vi "TAT_Start.vi"(8 "error In":errorcluster) -> ()   [LabVIEW 2017]
uses:
  <vilib>/addons/database/Connection.llb/Conn ObjectReference.ctl
  Controls/Ass. Loop Control.ctl
  <vilib>/addons/database/Connection.llb/DB Tools Open Connec (Path).vi
  <vilib>/addons/database/NI_Database_API.lvlib
panel:
  out "CYCLE COUNT STATION 2":string caption="CYCLE COUNT"
  out "RESULT STATION 2":bool caption="RESULT"
  out "BARCODE STATION 2":string caption="BARCODE"
  out "CYCLE STATUS STATION 2":string caption="CYCLE STATUS"
  out "PLC":bool
  in  "Stop":bool
  out "error out":errorcluster
  out "CYCLE COUNT STATION 1":string caption="CYCLE COUNT"
  out "BARCODE STATION 1":string caption="BARCODE"
  out "RESULT STATION 1":bool caption="RESULT"
  out "VARIENT":string
  out "USER":string
  in  "ASS-Alarms":bool
  in  "T-Alarms":bool
  out "CYCLE STATUS STATION 1":string caption="CYCLE STATUS"
  out "DATE/TIME":string
  # "RBC ORVM- TRACEABILITY, SCANNING & BARCODE PRINTING"
  # "STATION 1"
  # "STATION 2"
  # "Nm"
  # "REMAINING SQL CODE TO WRITE"
  # "KAPSE SONS ROBOTICS\n& AUTOMATION"
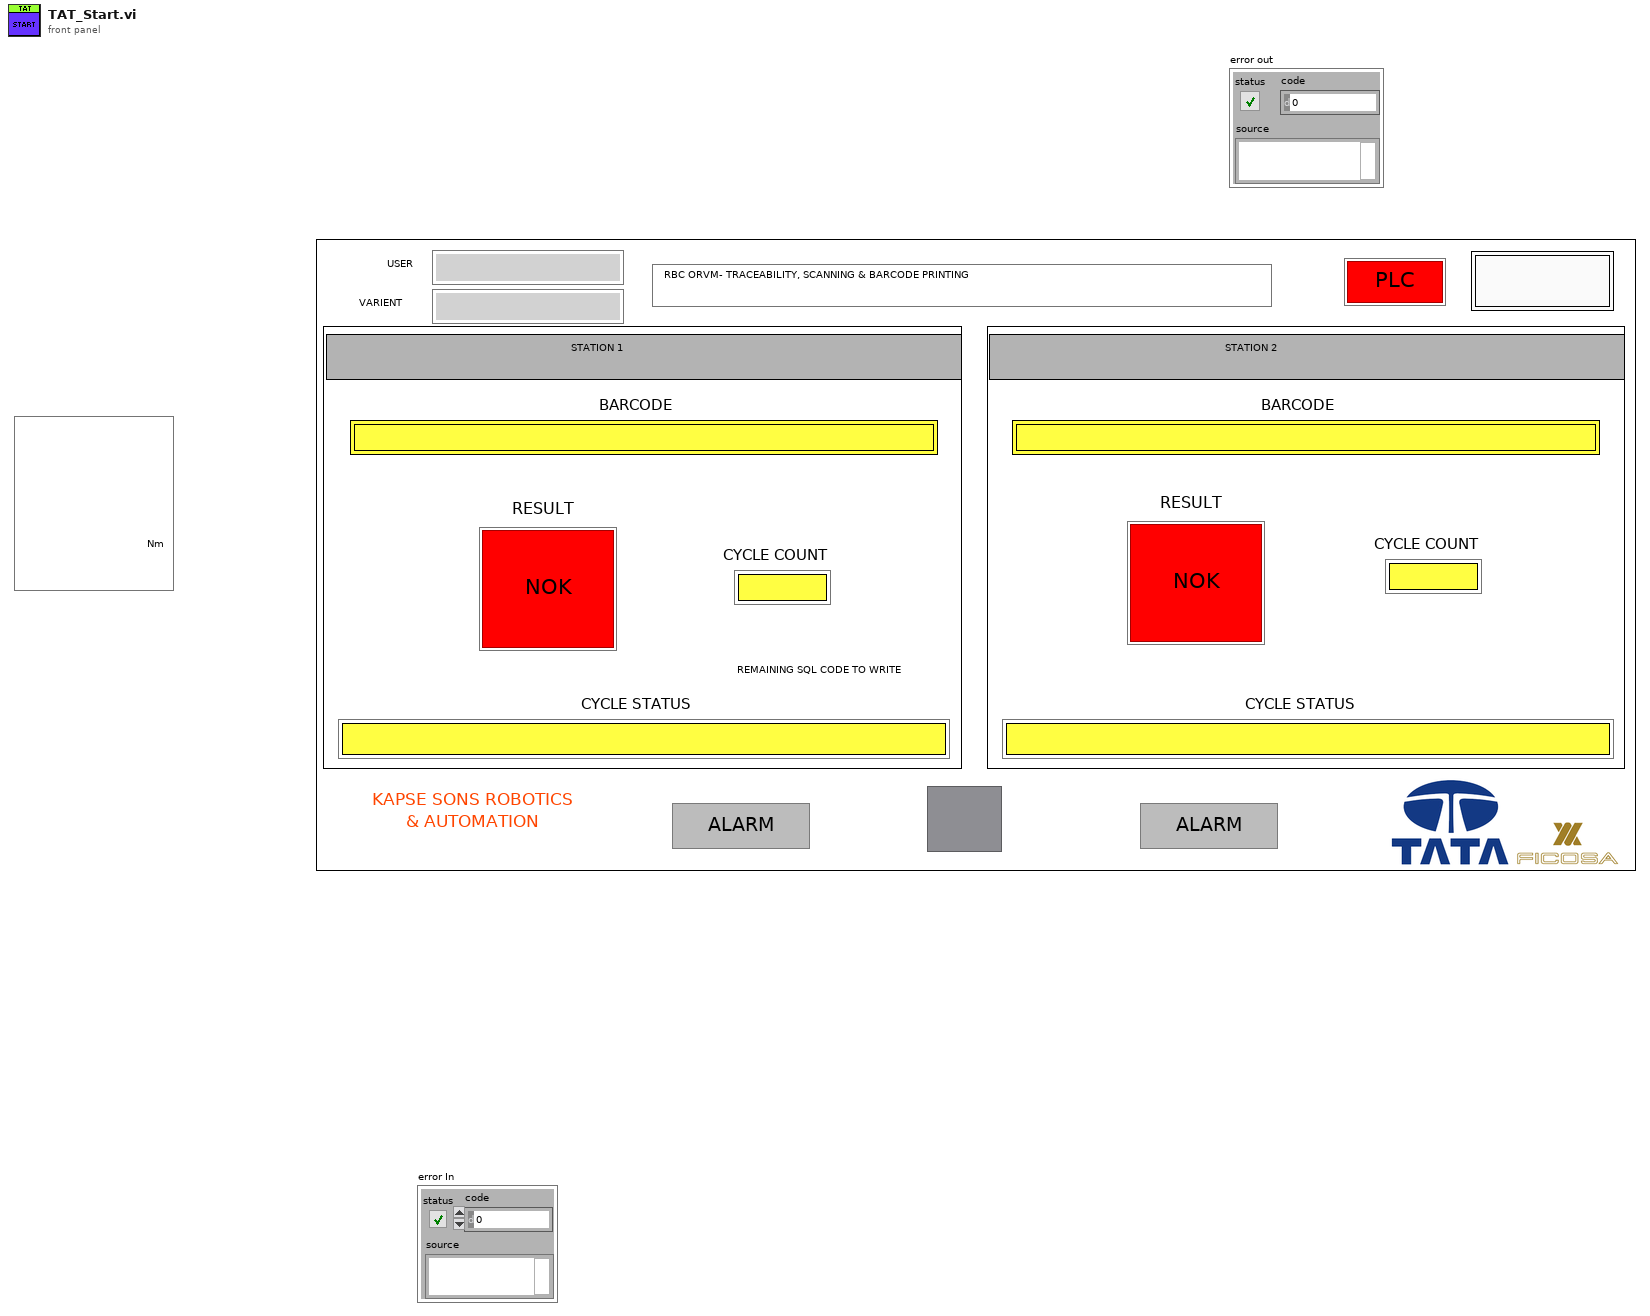
[diagram p1: front panel]
types:
  T1 = typedef "Ass. Loop Control.ctl" = enum16{"Cluster_update", "Waiting_for_scan", "barcode scan", "Int", "SaveReport ", "Barcode Print", "Start Cycle", "Wait", "Cycle End", "Stop"}
  T2 = typedef "NI_Database_API.lvlib/Conn ObjectReference.ctl" = refnum<k1>
  T3 = cluster{"Varient number":i32, "Varient name":string, "connection ID":refnum<k5>, "connection reference":T2, "Varient_Counter":u16}
  T4 = cluster{"Varient number":u16, "Varient name":string, "Barcode prefix":string, "connection ID":refnum<k5>, "connection reference":T2, "Batch_Size":u16}
  T5 = cluster{"seconds since 1Jan1904":timestamp, "Varient name":string, "BARCODE STATION 1":string, "table":string, "table":string}
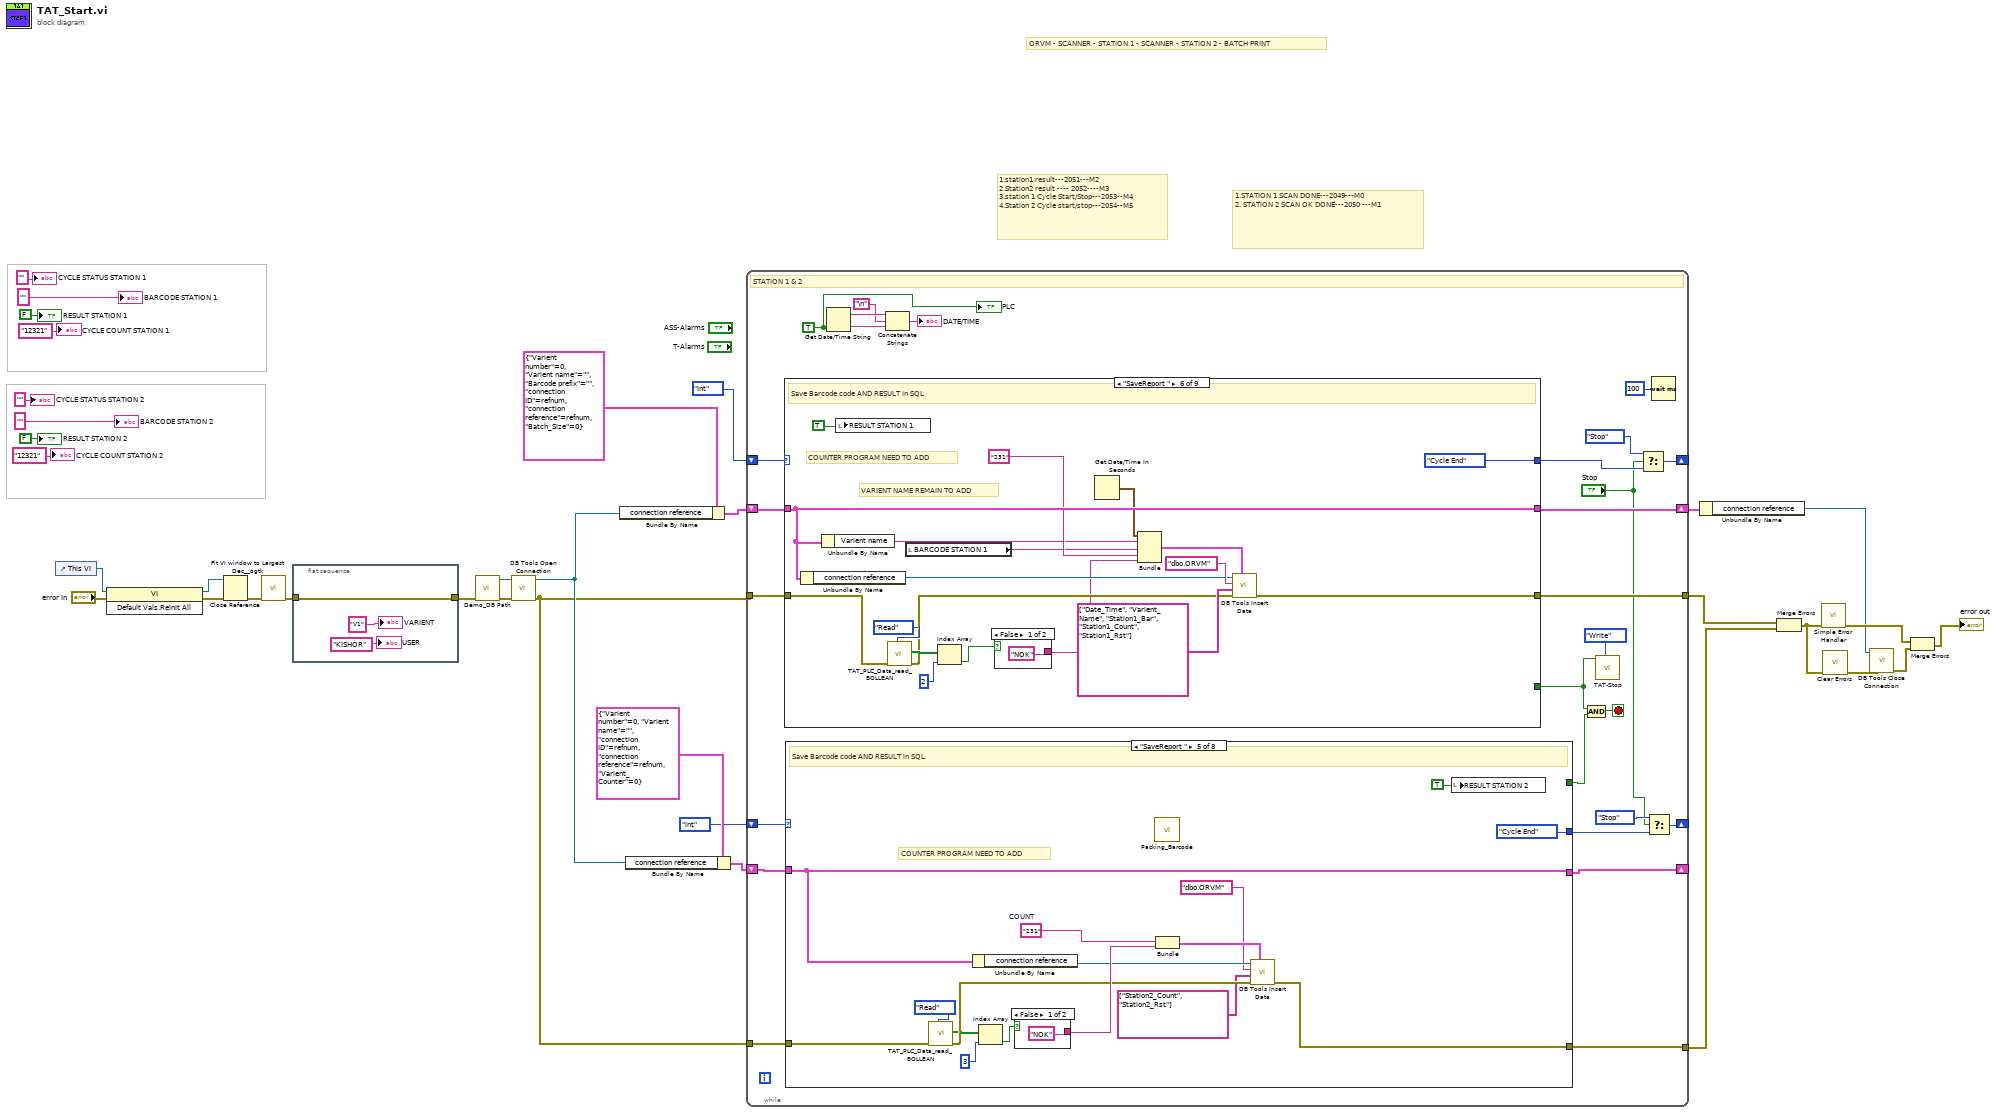
[diagram p0: block diagram]
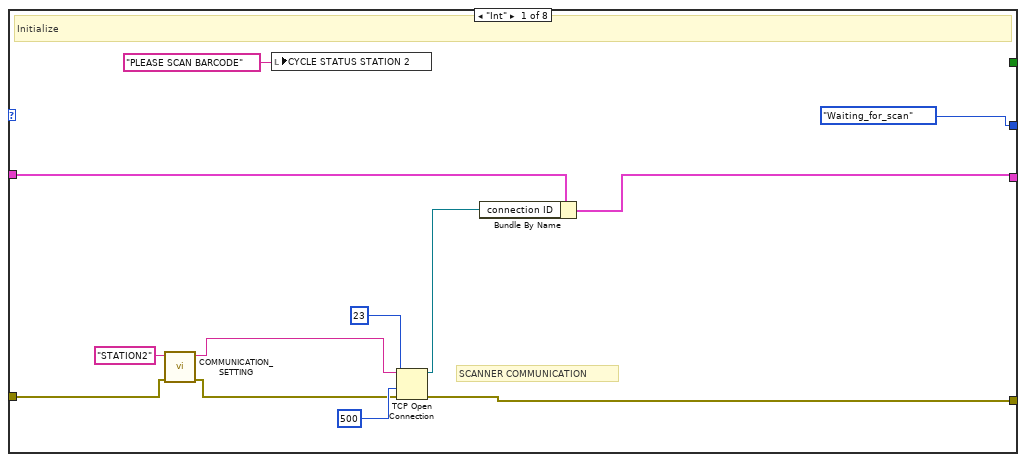
[diagram p2: hidden frame]
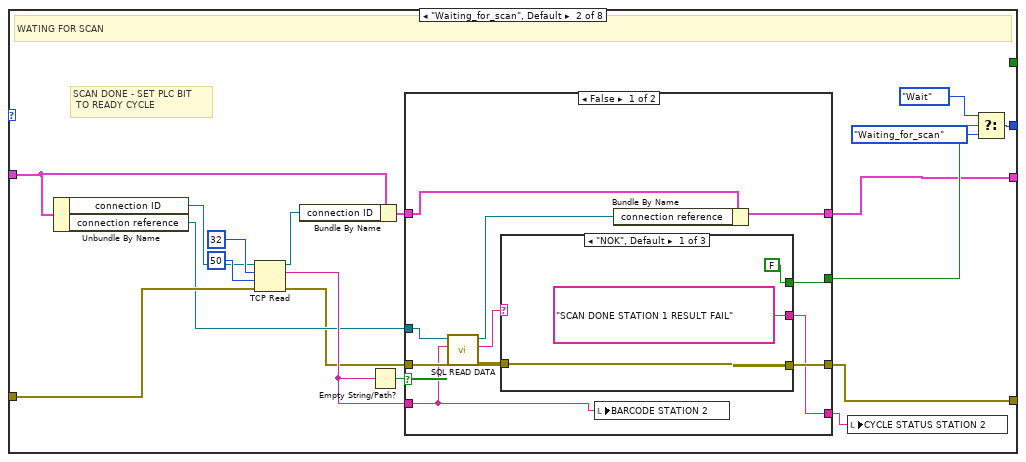
[diagram p3: hidden frame]
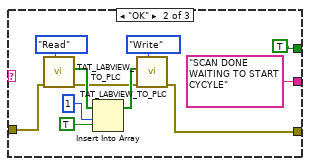
[diagram p4: hidden frame]
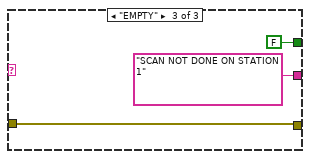
[diagram p5: hidden frame]
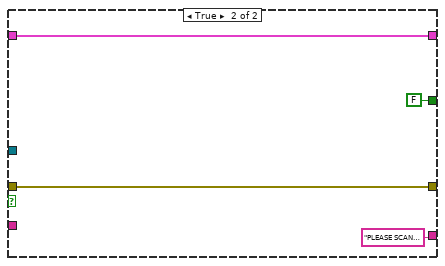
[diagram p6: hidden frame]
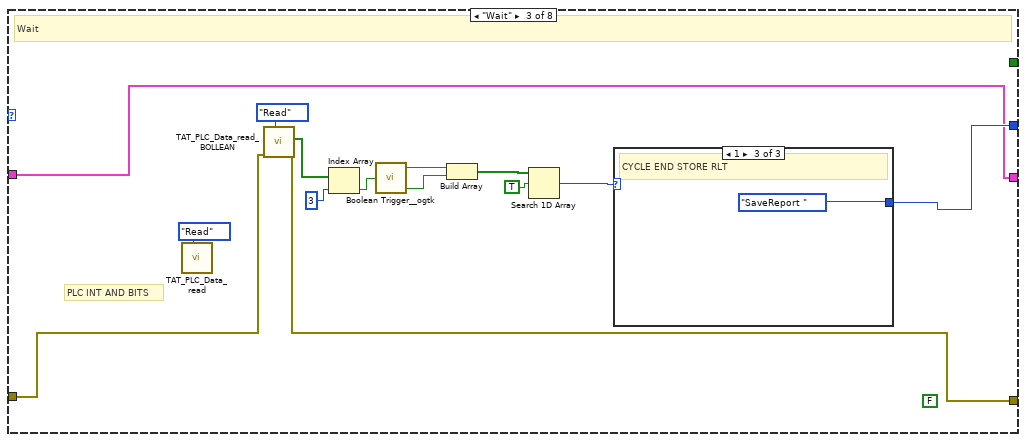
[diagram p7: hidden frame]
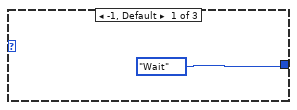
[diagram p8: hidden frame]
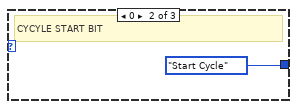
[diagram p9: hidden frame]
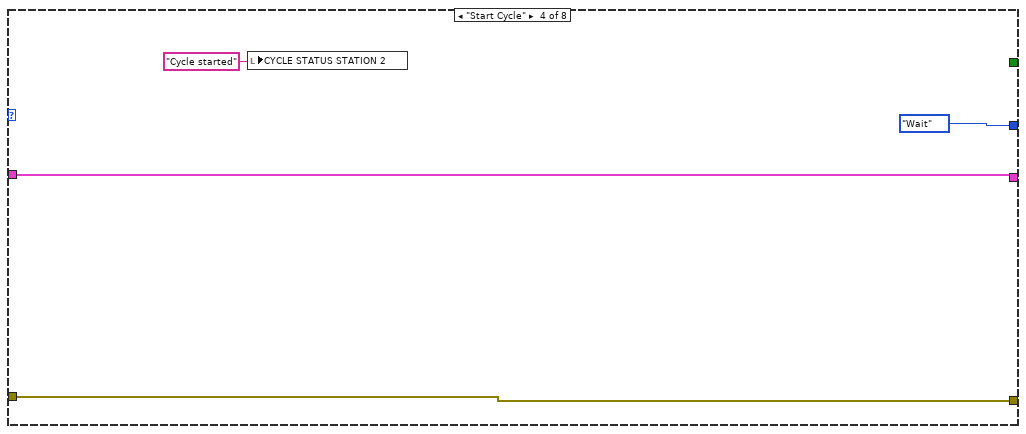
[diagram p10: hidden frame]
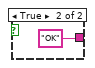
[diagram p11: hidden frame]
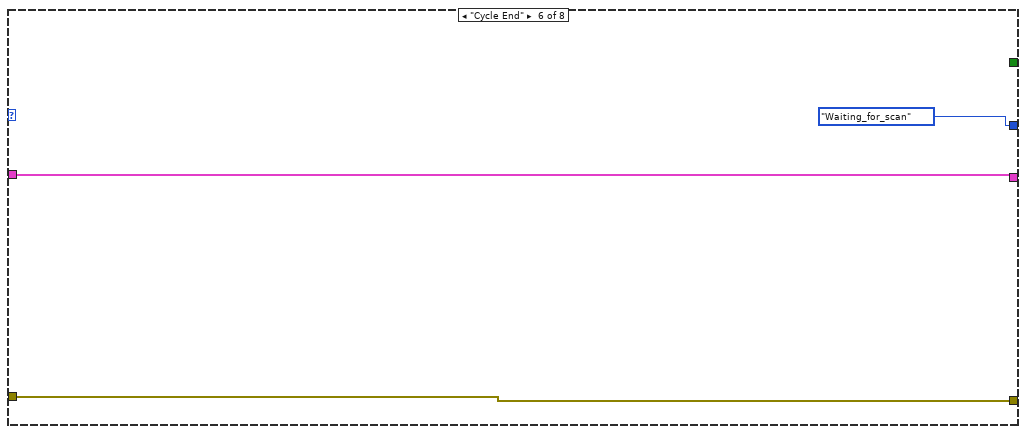
[diagram p12: hidden frame]
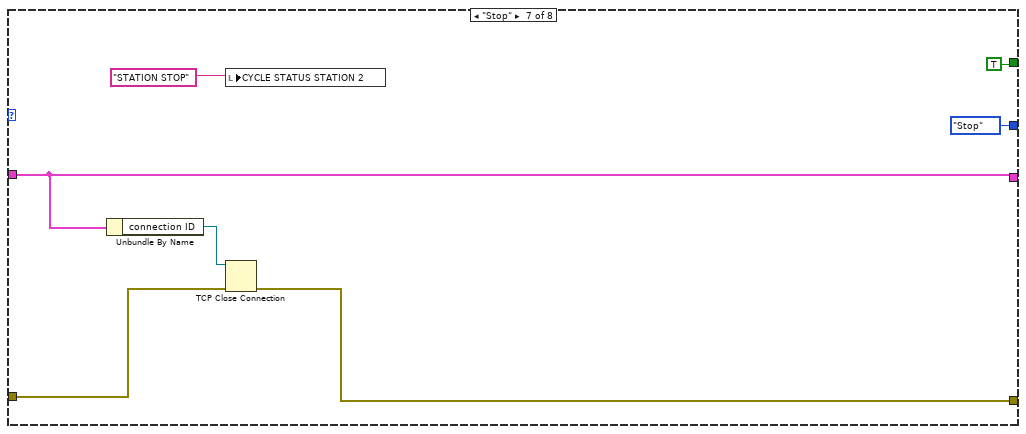
[diagram p13: hidden frame]
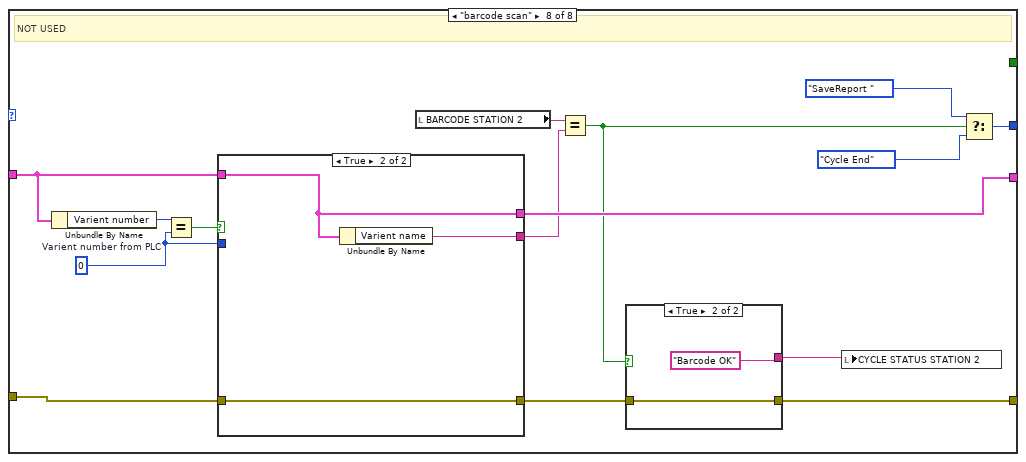
[diagram p14: hidden frame]
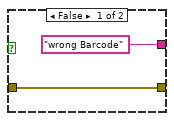
[diagram p15: hidden frame]
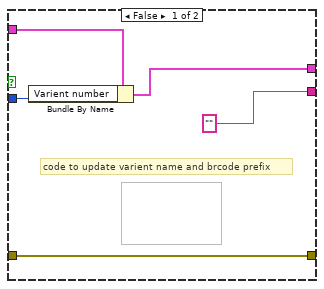
[diagram p16: hidden frame]
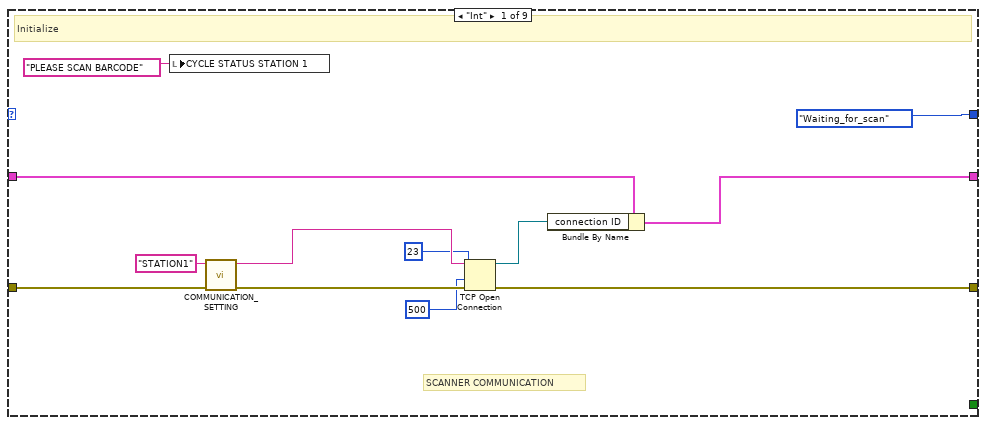
[diagram p17: hidden frame]
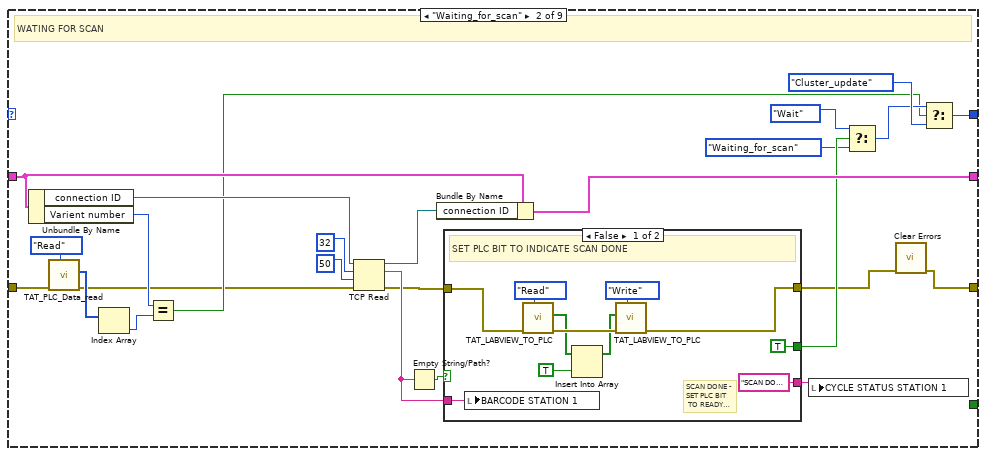
[diagram p18: hidden frame]
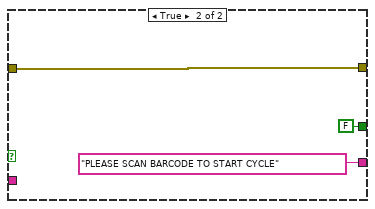
[diagram p19: hidden frame]
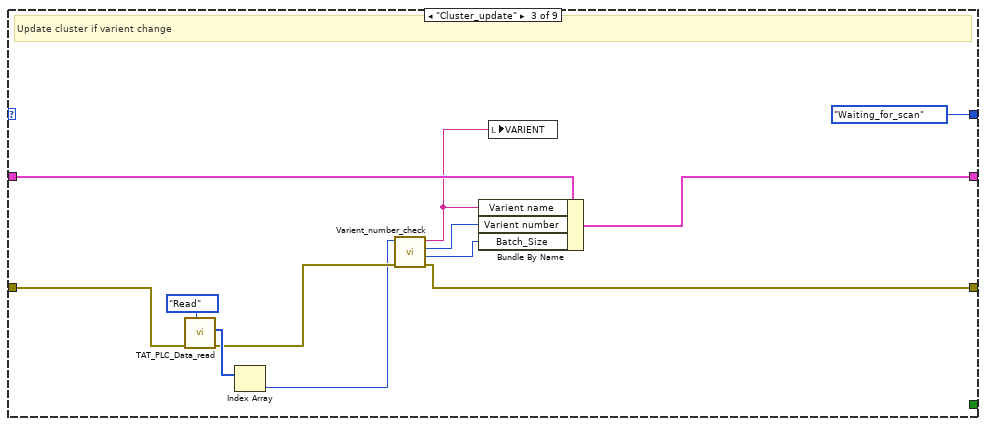
[diagram p20: hidden frame]
diagram:
  # "1.STATION 1 SCAN DONE---2049---M0\n2. STATION 2 SCAN OK DONE---2050 ---M1"
  # "1.station1 result---2051---M2\n2.Station2 result ---- 2052----M3\n3.station 1 Cycle Start/Stop---2053--M4\n4.Station 2 Cycle start/stop---2054--M5"
  # "ORVM - SCANNER - STATION 1 - SCANNER - STATION 2 - BATCH PRINT"
  n1 = control-ref of="This VI"() -> (w34:refnum<vi>)
  n2 = invoke class="VI" method="Default Vals.Reinit All"(reference=w34, error in="error In") -> (reference out=w31:refnum<vi>, error out=w32:errorcluster)  [unwired: 1 in, 1 out]
  n3 = Close Reference(reference=w31, error in (no error)=w32) -> (error out=w30:errorcluster)
  n4 = call <userlib>:"Fit VI window to Largest Dec__ogtk.vi"("error in (no error)"=w30) -> ("error out"=w29:errorcluster)  [unwired: 5 in, 1 out]
  n5 = flat-sequence {
    tunnel: [w37] -> w12
    tunnel: w29 -> [w37]
    frame #0 {
      "USER" <- "KISHOR"
      "VARIENT" <- "V1"
    }
  }
  n6 = call "Demo_DB Path.vi"("error in"=w12) -> ("error out"=w10:errorcluster, "DB Path"=w11:path)  [unwired: 9 in]
  n7 = call-poly <vilib>:"DB Tools Open Connection.vi"("error in (no error)"=w10, "connection information"=w11) -> ("error out"=w1:errorcluster, "connection reference"=w9:T2)  [unwired: 6 in]
  n8 = Bundle By Name(cluster=T4 {"Varient number"=0, "Varient name"="", "Barcode prefix"="", "connection ID"=refnum, "connection reference"=refnum, "Batch_Size"=0}, "connection reference"=w9) -> (w22:T4)
  n9 = Bundle By Name(cluster=T3 {"Varient number"=0, "Varient name"="", "connection ID"=refnum, "connection reference"=refnum, "Varient_Counter"=0}, "connection reference"=w9) -> (w20:T3)
  n10 = while {
    tunnel: w1 -> [w59]
    shift-right: [w58] -> _
    shift-left: Ass._Loop_Control."Int" ("Enum") -> [w64]
    shift-right: [w62] -> w3
    shift-left: w22 -> [w61]
    tunnel: [w60] -> w24
    tunnel: w1 -> [w50]
    tunnel: [w49] -> w13
    shift-right: [w46] -> _
    shift-left: w20 -> [w48]
    shift-right: [w43] -> _
    shift-left: Ass._Loop_Control."Int" ("Enum") -> [w47]
    stop <- w41 stop-if-true
    w51 = TRUE ("want seconds? (F)")
    # "STATION 1 & 2"
    n11 = case shown="\"SaveReport \"" w64 {
      tunnel: [Ass._Loop_Control."Waiting_for_scan" ("Enum") w218 Ass._Loop_Control."Waiting_for_scan" ("Enum") w273 Ass._Loop_Control."Wait" ("Enum") Ass._Loop_Control."Cycle End" ("Enum") Ass._Loop_Control."Waiting_for_scan" ("Enum") Ass._Loop_Control."Stop" ("Enum") w323] -> w57
      tunnel: [w206 w232 w257 w275 w287 w304 w311 w314 w329] -> w62
      tunnel: w61 -> [w207 w233 w258 w275 w287 w304 w311 w314 w330]
      tunnel: [_ _ _ FALSE _ _ _ TRUE _] -> w38
      tunnel: [w203 w226 w264 w267 w284 w299 w310 w315 w321] -> w60
      tunnel: w59 -> [w204 w223 w261 w268 w284 w288 w310 w316 w332]
      frame "Int" {
        # "SCANNER COMMUNICATION"
        # "Initialize"
        n12 = local write "CYCLE STATUS STATION 1"("PLEASE SCAN BARCODE" ("Cycle Status")) -> ()
        n13 = call "COMMUNICATION_SETTING.vi"("error in"=w204, "STATION"="STATION1") -> ("error out"=w212:errorcluster, "COM"=w210:string)  [unwired: 8 in]
        n14 = TCP Open Connection(address=w210, remote port or service name=u16 23, timeout ms (60000)=500, error in (no error)=w212) -> (connection ID=w205:refnum<k5>, error out=w203:errorcluster)  [unwired: 1 in]
        n15 = Bundle By Name(cluster=w207, "connection ID"=w205) -> (w206:T4)
      }
      frame "Waiting_for_scan" {
        # "WATING FOR SCAN"
        n16 = Unbundle By Name(w233) -> ("connection ID"=w235:refnum<k5>, "Varient number"=w222:u16)
        n17 = call "TAT_PLC_Data_read.vi"("Enum"=enum16{"Read", "Write"}."Read", "error in (no error)"=w223) -> ("error out"=w216:errorcluster, "Array 2"=w225:u16[])  [unwired: 8 in]
        n18 = Index Array(array=w225) -> (element=w215:u16)  [unwired: 1 in]
        n19 = Equal?(x=w222, y=w215) -> (x = y?=w217:bool)
        n20 = TCP Read(connection ID=w235, bytes to read=32, error in (no error)=w216, 9:50 ("timeout ms (25000)")) -> (connection ID out=w234:refnum<k5>, data out=w237:string, error out=w228:errorcluster)  [unwired: 1 in]
        n21 = Empty String/Path?(string/path=w237) -> (empty?=w236:bool)
        n22 = Bundle By Name(cluster=w233, "connection ID"=w234) -> (w232:T4)
        n23 = case shown="False" w236 {
          tunnel: w237 -> [w240 _]
          tunnel: [TRUE FALSE] -> w231
          tunnel: ["SCAN DONE WAITING TO START CYCYLE" ("Cycle Status") "PLEASE SCAN BARCODE TO START CYCLE" ("Cycle Status")] -> w229
          tunnel: w228 -> [w245 w251]
          tunnel: [w248 w251] -> w227
          frame False {
            # "SCAN DONE - SET PLC BIT\n TO READY CYCLE"
            # "SET PLC BIT TO INDICATE SCAN DONE"
            n24 = local write "BARCODE STATION 1"(w240) -> ()
            n25 = call "TAT_LABVIEW_TO_PLC.vi"("Enum"=enum16{"Read", "Write"}."Read", "error in (no error)"=w245) -> ("error out"=w244:errorcluster, "Array 2"=w243:bool[])  [unwired: 8 in]
            n26 = Insert Into Array(array=w243, new element=TRUE) -> (w242:bool[])  [unwired: 1 in]
            n27 = call "TAT_LABVIEW_TO_PLC.vi"("Enum"=enum16{"Read", "Write"}."Write", "error in (no error)"=w244, "Array"=w242) -> ("error out"=w248:errorcluster)  [unwired: 7 in, 1 out]
          }
          frame True {
          }
        }
        n28 = local write "CYCLE STATUS STATION 1"(w229) -> ()
        n29 = Select(t=Ass._Loop_Control."Wait" ("Enum"), s=w231, f=Ass._Loop_Control."Waiting_for_scan" ("Enum")) -> (s? t:f=w219:T1)
        n30 = call <vilib>:"Clear Errors.vi"("error in (no error)"=w227) -> ("error out"=w226:errorcluster)  [unwired: 5 in, 1 out]
        n31 = Select(t=w219, s=w217, f=Ass._Loop_Control."Cluster_update" ("Enum")) -> (s? t:f=w218:T1)
      }
      frame "Cluster_update" {
        # "Update cluster if varient change"
        n32 = call "TAT_PLC_Data_read.vi"("Enum"=enum16{"Read", "Write"}."Read", "error in (no error)"=w261) -> ("error out"=w255:errorcluster, "Array 2"=w263:u16[])  [unwired: 8 in]
        n33 = Index Array(array=w263) -> (element=w254:u16)  [unwired: 1 in]
        n34 = call "Varient_number_check.vi"("error in"=w255, "Varient No."=w254) -> ("error out"=w264:errorcluster, "Batch Size"=w259:i32, "Varient Number"=w260:i32, "Varient Name"=w256:string)  [unwired: 6 in]
        n35 = Bundle By Name(cluster=w258, "Varient name"=w256, "Varient number"=w260, "Batch_Size"=w259) -> (w257:T4)
        n36 = local write "VARIENT"(w256) -> ()
      }
      frame "Wait", Default {
        # "Wait"
        n37 = disable-structure shown="Disabled" {
          frame Disabled {
            # "PLC INT AND BITS"
            n38 = call "TAT_PLC_Data_read.vi"("Enum"=enum16{"Read", "Write"}."Read") -> ()  [unwired: 9 in, 2 out]
          }
          frame Enabled {
          }
        }
        n39 = call "TAT_PLC_Data_read_BOLLEAN.vi"("Enum"=enum16{"Read", "Write"}."Read", "error in (no error)"=w268) -> ("error out"=w267:errorcluster, "Array 2"=w269:bool[])  [unwired: 8 in]
        n40 = Index Array(array=w269, index=2) -> (element=w270:bool)
        n41 = call <userlib>:"Boolean Trigger__ogtk.vi"("Boolean Input"=w270) -> ("Rising Edge"=w278:bool, "Falling Edge"=w276:bool)  [unwired: 1 in]
        n42 = Build Array(w278, w276) -> (w277:bool[])
        n43 = Search 1D Array(1D array=w277, element=TRUE ("Boolean Input")) -> (index of element=w274:i32)  [unwired: 1 in]
        n44 = case shown="1" w274 {
          tunnel: [Ass._Loop_Control."Wait" ("Enum") Ass._Loop_Control."Start Cycle" ("Enum") Ass._Loop_Control."SaveReport " ("Enum")] -> w273
          frame -1, Default {
          }
          frame 0 {
            # "CYCYLE START BIT"
          }
          frame 1 {
            # "CYCLE END STORE RLT"
          }
        }
      }
      frame "Start Cycle" {
        n45 = local write "CYCLE STATUS STATION 1"("Cycle started" ("Cycle Status")) -> ()
      }
      frame "SaveReport " {
        # "COUNTER PROGRAM NEED TO ADD"
        # "VARIENT NAME REMAIN TO ADD"
        # "Save Barcode code AND RESULT in SQL"
        n46 = Unbundle By Name(w304) -> ("connection reference"=w298:T2)
        n47 = Unbundle By Name(w304) -> ("Varient name"=w295:string)
        n48 = local write "RESULT STATION 1"(TRUE) -> ()
        n49 = call "TAT_PLC_Data_read_BOLLEAN.vi"("Enum"=enum16{"Read", "Write"}."Read", "error in (no error)"=w288) -> ("error out"=w292:errorcluster, "Array 2"=w293:bool[])  [unwired: 8 in]
        n50 = local read "BARCODE STATION 1"() -> (w296:string)
        n51 = Index Array(array=w293, index=2) -> (element=w289:bool)
        n52 = case shown="False" w289 {
          tunnel: ["NOK" ("table") "OK" ("table")] -> w290
          frame False {
          }
          frame True {
          }
        }
        n53 = Get Date/Time In Seconds() -> (seconds since 1Jan1904=w297:timestamp)
        n54 = Bundle("seconds since 1Jan1904"=w297, "Varient name"=w295, "BARCODE STATION 1"=w296, "table"="231", "table"=w290) -> (w302:T5)  [unwired: 1 in]
        n55 = call <vilib>:"DB Tools Insert Data.vi"("data"=w302, "error in (no error)"=w292, "columns"=string[] ["Date_Time", "Varient_Name", "Station1_Bar", "Station1_Count", "Station1_Rst"] ("columns 2"), "table"="dbo.ORVM", "connection reference"=w298) -> ("error out"=w299:errorcluster)  [unwired: 5 in, 1 out]
      }
      frame "Cycle End" {
      }
      frame "Stop" {
        n56 = local write "CYCLE STATUS STATION 1"("STATION STOP" ("Cycle Status")) -> ()
        n57 = Unbundle By Name(w314) -> ("connection ID"=w313:refnum<k5>)
        n58 = TCP Close Connection(connection ID=w313, error in (no error)=w316) -> (error out=w315:errorcluster)  [unwired: 1 in, 1 out]
      }
      frame "barcode scan" {
        w328 = 0  # Varient number from PLC
        # "NOT USED"
        n59 = Unbundle By Name(w330) -> ("Varient number"=w333:u16)
        n60 = Equal?(x=w333, y=w328) -> (x = y?=w331:bool)
        n61 = case shown="True" w331 {
          tunnel: [w342 w345] -> w322
          tunnel: w332 -> [w342 w345]
          tunnel: [w340 w344] -> w329
          tunnel: w330 -> [w341 w344]
          tunnel: w328 -> [w339 _]
          tunnel: ["" ("Barcode prefix") w343] -> w326
          frame False {
            # "code to update varient name and brcode prefix"
            n62 = Bundle By Name(cluster=w341, "Varient number"=w339) -> (w340:T4)
          }
          frame True {
            n63 = Unbundle By Name(w344) -> ("Barcode prefix"=w343:string)
          }
        }
        n64 = local read "BARCODE STATION 1"() -> (w327:string)
        n65 = Equal?(x=w327, y=w326) -> (x = y?=w319:bool)
        n66 = case shown="True" w319 {
          tunnel: [w335 w337] -> w321
          tunnel: w322 -> [w335 w337]
          tunnel: ["wrong Barcode" ("Cycle Status") "Barcode OK" ("Cycle Status")] -> w320
          frame False {
          }
          frame True {
          }
        }
        n67 = Select(t=Ass._Loop_Control."SaveReport " ("Enum"), s=w319, f=Ass._Loop_Control."Cycle End" ("Enum")) -> (s? t:f=w323:T1)
        n68 = local write "CYCLE STATUS STATION 1"(w320) -> ()
      }
    }
    n69 = case shown="\"SaveReport \"" w47 {
      tunnel: [Ass._Loop_Control."Waiting_for_scan" ("Enum") w86 w135 Ass._Loop_Control."Wait" ("Enum") Ass._Loop_Control."Cycle End" ("Enum") Ass._Loop_Control."Waiting_for_scan" ("Enum") Ass._Loop_Control."Stop" ("Enum") w182] -> w44
      tunnel: [w65 w77 w130 w144 w148 w166 w172 w188] -> w46
      tunnel: [w68 w80 w128 w145 w150 w168 w173 w180] -> w49
      tunnel: w50 -> [w74 w90 w129 w145 w149 w168 w174 w190]
      tunnel: w48 -> [w66 w83 w130 w144 w148 w166 w172 w177]
      tunnel: [_ _ _ _ _ _ TRUE _] -> w40
      frame "Int" {
        # "SCANNER COMMUNICATION"
        # "Initialize"
        n70 = call "COMMUNICATION_SETTING.vi"("error in"=w74, "STATION"="STATION2") -> ("error out"=w69:errorcluster, "COM"=w71:string)  [unwired: 8 in]
        n71 = local write "CYCLE STATUS STATION 2"("PLEASE SCAN BARCODE" ("Cycle Status")) -> ()
        n72 = TCP Open Connection(address=w71, remote port or service name=u16 23, timeout ms (60000)=500, error in (no error)=w69) -> (connection ID=w67:refnum<k5>, error out=w68:errorcluster)  [unwired: 1 in]
        n73 = Bundle By Name(cluster=w66, "connection ID"=w67) -> (w65:T3)
      }
      frame "Waiting_for_scan", Default {
        # "SCAN DONE - SET PLC BIT\n TO READY CYCLE"
        # "WATING FOR SCAN"
        n74 = Unbundle By Name(w83) -> ("connection ID"=w82:refnum<k5>, "connection reference"=w81:T2)
        n75 = TCP Read(connection ID=w82, bytes to read=32, error in (no error)=w90, 9:50 ("timeout ms (25000)")) -> (connection ID out=w89:refnum<k5>, data out=w92:string, error out=w79:errorcluster)  [unwired: 1 in]
        n76 = Bundle By Name(cluster=w83, "connection ID"=w89) -> (w78:T3)
        n77 = Empty String/Path?(string/path=w92) -> (empty?=w91:bool)
        n78 = case shown="False" w91 {
          tunnel: w92 -> [w95 _]
          tunnel: [w96 FALSE] -> w88
          tunnel: [w97 "PLEASE SCAN BARCODE TO START CYCLE" ("Cycle Status")] -> w84
          tunnel: w81 -> [w103 _]
          tunnel: [w99 w124] -> w80
          tunnel: w79 -> [w101 w124]
          tunnel: [w105 w123] -> w77
          tunnel: w78 -> [w104 w123]
          frame False {
            n79 = call "SQL READ DATA.vi"("error out 2"=w101, "Barcode"=w95, "connection reference"=w103) -> ("error out"=w100:errorcluster, "Station1_Rst"=w98:string, "connection reference out"=w102:T2)  [unwired: 6 in]
            n80 = case shown="\"NOK\", Default" w98 {
              tunnel: [w108 w109 w122] -> w99
              tunnel: w100 -> [w108 w110 w122]
              tunnel: ["SCAN DONE STATION 1 RESULT FAIL" ("Cycle Status") "SCAN DONE WAITING TO START CYCYLE" ("Cycle Status") "SCAN NOT DONE ON STATION 1" ("Cycle Status")] -> w97
              tunnel: [FALSE TRUE FALSE] -> w96
              frame "NOK", Default {
              }
              frame "OK" {
                n81 = call "TAT_LABVIEW_TO_PLC.vi"("Enum"=enum16{"Read", "Write"}."Read", "error in (no error)"=w110) -> ("error out"=w115:errorcluster, "Array 2"=w116:bool[])  [unwired: 8 in]
                n82 = Insert Into Array(array=w116, index=1, new element=TRUE) -> (w117:bool[])
                n83 = call "TAT_LABVIEW_TO_PLC.vi"("Enum"=enum16{"Read", "Write"}."Write", "error in (no error)"=w115, "Array"=w117) -> ("error out"=w109:errorcluster)  [unwired: 7 in, 1 out]
              }
              frame "EMPTY" {
              }
            }
            n84 = local write "BARCODE STATION 2"(w95) -> ()
            n85 = Bundle By Name(cluster=w104, "connection reference"=w102) -> (w105:T3)
          }
          frame True {
          }
        }
        n86 = local write "CYCLE STATUS STATION 2"(w84) -> ()
        n87 = Select(t=Ass._Loop_Control."Wait" ("Enum"), s=w88, f=Ass._Loop_Control."Waiting_for_scan" ("Enum")) -> (s? t:f=w86:T1)
      }
      frame "Wait" {
        (unwired) FALSE
        # "PLC INT AND BITS"
        # "Wait"
        n88 = call "TAT_PLC_Data_read.vi"("Enum"=enum16{"Read", "Write"}."Read") -> ()  [unwired: 9 in, 2 out]
        n89 = call "TAT_PLC_Data_read_BOLLEAN.vi"("Enum"=enum16{"Read", "Write"}."Read", "error in (no error)"=w129) -> ("error out"=w128:errorcluster, "Array 2"=w131:bool[])  [unwired: 8 in]
        n90 = Index Array(array=w131, index=3) -> (element=w132:bool)
        n91 = call <userlib>:"Boolean Trigger__ogtk.vi"("Boolean Input"=w132) -> ("Rising Edge"=w139:bool, "Falling Edge"=w137:bool)  [unwired: 1 in]
        n92 = Build Array(w139, w137) -> (w138:bool[])
        n93 = Search 1D Array(1D array=w138, element=TRUE ("Boolean Input")) -> (index of element=w136:i32)  [unwired: 1 in]
        n94 = case shown="1" w136 {
          tunnel: [Ass._Loop_Control."Wait" ("Enum") Ass._Loop_Control."Start Cycle" ("Enum") Ass._Loop_Control."SaveReport " ("Enum")] -> w135
          frame -1, Default {
          }
          frame 0 {
            # "CYCYLE START BIT"
          }
          frame 1 {
            # "CYCLE END STORE RLT"
          }
        }
      }
      frame "Start Cycle" {
        n95 = local write "CYCLE STATUS STATION 2"("Cycle started" ("Cycle Status")) -> ()
      }
      frame "SaveReport " {
        w153 = "231"  # COUNT
        # "COUNTER PROGRAM NEED TO ADD"
        # "Save Barcode code AND RESULT in SQL"
        n96 = call "TAT_PLC_Data_read_BOLLEAN.vi"("Enum"=enum16{"Read", "Write"}."Read", "error in (no error)"=w149) -> ("error out"=w158:errorcluster, "Array 2"=w157:bool[])  [unwired: 8 in]
        n97 = Unbundle By Name(w148) -> ("connection reference"=w155:T2)
        n98 = Index Array(array=w157, index=3) -> (element=w161:bool)
        n99 = case shown="False" w161 {
          tunnel: ["NOK" ("table") "OK" ("table")] -> w160
          frame False {
          }
          frame True {
          }
        }
        n100 = call "Packing_Barcode.vi"() -> ()  [unwired: 11 in, 1 out]
        n101 = Bundle("COUNT"=w153, "table"=w160) -> (w152:cluster{"COUNT":string, "table":string})  [unwired: 1 in]
        n102 = call <vilib>:"DB Tools Insert Data.vi"("data"=w152, "error in (no error)"=w158, "columns"=string[] ["Station2_Count", "Station2_Rst"] ("columns 2"), "table"="dbo.ORVM", "connection reference"=w155) -> ("error out"=w150:errorcluster)  [unwired: 5 in, 1 out]
        n103 = local write "RESULT STATION 2"(TRUE) -> ()
      }
      frame "Cycle End" {
      }
      frame "Stop" {
        n104 = Unbundle By Name(w172) -> ("connection ID"=w171:refnum<k5>)
        n105 = local write "CYCLE STATUS STATION 2"("STATION STOP" ("Cycle Status")) -> ()
        n106 = TCP Close Connection(connection ID=w171, error in (no error)=w174) -> (error out=w173:errorcluster)  [unwired: 1 in, 1 out]
      }
      frame "barcode scan" {
        w187 = 0  # Varient number from PLC
        # "NOT USED"
        n107 = Unbundle By Name(w177) -> ("Varient number"=w176:i32)
        n108 = Equal?(x=w176, y=w187) -> (x = y?=w189:bool)
        n109 = case shown="True" w189 {
          tunnel: [w199 w202] -> w181
          tunnel: w190 -> [w199 w202]
          tunnel: [w198 w200] -> w188
          tunnel: w187 -> [w197 _]
          tunnel: ["" ("Barcode prefix") w201] -> w185
          tunnel: w177 -> [w195 w200]
          frame False {
            # "code to update varient name and brcode prefix"
            n110 = Bundle By Name(cluster=w195, "Varient number"=w197) -> (w198:T3)
          }
          frame True {
            n111 = Unbundle By Name(w200) -> ("Varient name"=w201:string)
          }
        }
        n112 = local read "BARCODE STATION 2"() -> (w186:string)
        n113 = Equal?(x=w186, y=w185) -> (x = y?=w178:bool)
        n114 = case shown="True" w178 {
          tunnel: [w192 w194] -> w180
          tunnel: w181 -> [w192 w194]
          tunnel: ["wrong Barcode" ("Cycle Status") "Barcode OK" ("Cycle Status")] -> w179
          frame False {
          }
          frame True {
          }
        }
        n115 = local write "CYCLE STATUS STATION 2"(w179) -> ()
        n116 = Select(t=Ass._Loop_Control."SaveReport " ("Enum"), s=w178, f=Ass._Loop_Control."Cycle End" ("Enum")) -> (s? t:f=w182:T1)
      }
    }
    n117 = Get Date/Time String(want seconds? (F)=w51) -> (date string=w54:string, time string=w53:string)  [unwired: 2 in]
    n118 = Concatenate Strings(w54, "\n", w53) -> (→"DATE/TIME":string)
    n119 = And(x=w38, y=w40) -> (x .and. y?=w41:bool)
    n120 = call "TAT-Stop.vi"("Enum"=enum16{"Read", "Write"}."Write", "Stop"=w38) -> ()  [unwired: 9 in, 1 out]
    n121 = Select(t=Ass._Loop_Control."Stop" ("Enum"), s="Stop", f=w57) -> (s? t:f=w58:T1)
    n122 = Select(t=Ass._Loop_Control."Stop" ("Enum"), s="Stop", f=w44) -> (s? t:f=w43:T1)
    n123 = Wait (ms)(milliseconds to wait=u32 100) -> ()  [unwired: 1 out]
    "PLC" <- w51
  }
  n124 = Unbundle By Name(w3) -> ("connection reference"=w2:T2)
  n125 = Merge Errors(w24, w13) -> (w8:errorcluster)
  n126 = call <vilib>:"Simple Error Handler.vi"("error in (no error)"=w8) -> ("error out"=w5:errorcluster)  [unwired: 4 in, 4 out]
  n127 = call <vilib>:"Clear Errors.vi"("error in (no error)"=w8) -> ("error out"=w7:errorcluster)  [unwired: 5 in, 1 out]
  n128 = call <vilib>:"DB Tools Close Connection.vi"("error in (no error)"=w7, "connection reference"=w2) -> ("error out"=w6:errorcluster)  [unwired: 5 in]
  n129 = Merge Errors(w5, w6) -> (→"error out":errorcluster)
  "CYCLE STATUS STATION 1" <- ""
  "BARCODE STATION 1" <- ""
  "CYCLE COUNT STATION 1" <- "12321"
  "CYCLE STATUS STATION 2" <- ""
  "BARCODE STATION 2" <- ""
  "RESULT STATION 1" <- FALSE ("want seconds? (F)")
  "RESULT STATION 2" <- FALSE ("want seconds? (F)")
  "CYCLE COUNT STATION 2" <- "12321"
